vi "Triangle.vi"() -> ()   [LabVIEW 2017]
panel:
  out "Numeric":i32
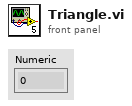
[diagram p1: front panel]
types:
  T1 = enum16{"Full", "Half", "Quarter", "Eighth", "Sixteenth"}
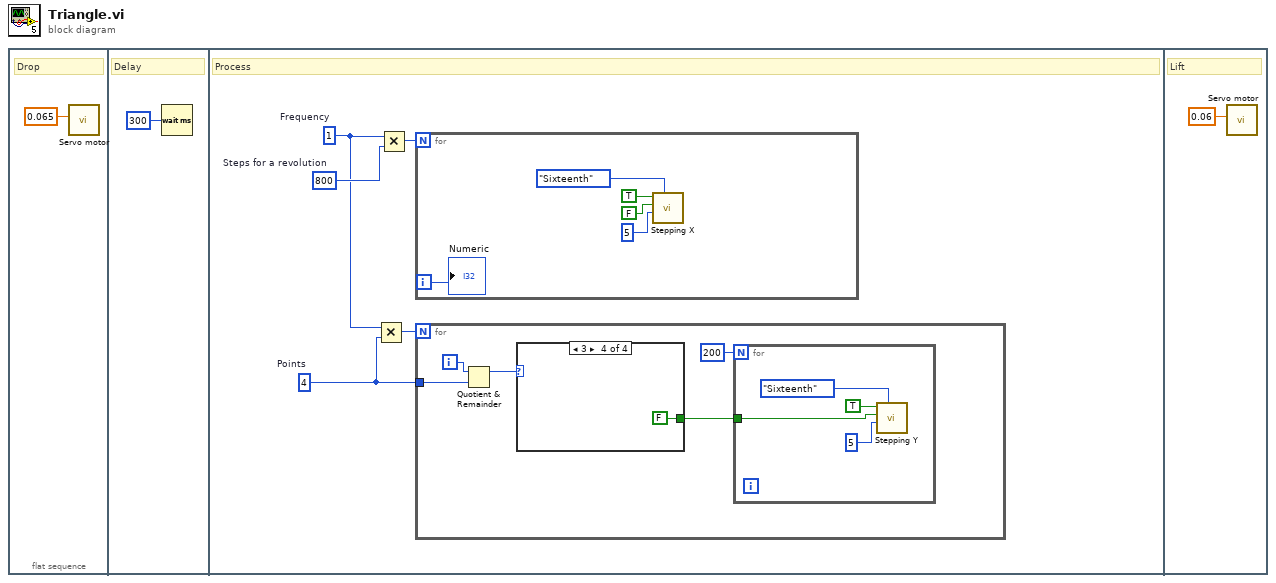
[diagram p0: block diagram]
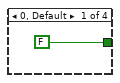
[diagram p2: hidden frame]
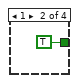
[diagram p3: hidden frame]
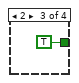
[diagram p4: hidden frame]
diagram:
  n1 = flat-sequence {
    frame #0 {
      # "Drop"
      n2 = call "Servo motor.vi"("Duty Cycle"=0.065) -> ()  [unwired: 9 in, 2 out]
    }
    frame #1 {
      # "Delay"
      n3 = Wait (ms)(milliseconds to wait=u32 300) -> ()  [unwired: 1 out]
    }
    frame #2 {
      w3 = 4  # Points
      w4 = 1  # Frequency
      w5 = 800  # Steps for a revolution
      # "Process"
      n4 = Multiply(x=w4, y=w3) -> (x*y=w7:i32)
      n5 = Multiply(x=w4, y=w5) -> (x*y=w6:i32)
      n6 = for {
        N: w6 -> [_]
        i -> [w25]
        n7 = call "Stepping X.vi"("Microstep size"=T1."Sixteenth", "Speed"=u32 5, "Direction"=FALSE, "Enable"=TRUE) -> ()  [unwired: 7 in, 1 out]
        "Numeric" <- w25
      }
      n8 = for {
        N: w7 -> [_]
        tunnel: w3 -> [w11]
        i -> [w12]
        n9 = Quotient & Remainder(x=w12, y=w11) -> (x-y*floor(x/y)=w10:i32)  [unwired: 1 out]
        n10 = case shown="3" w10 {
          tunnel: [FALSE ("Direction") TRUE ("Direction") TRUE ("Direction") FALSE ("Direction")] -> w9
          frame 0, Default {
          }
          frame 1 {
          }
          frame 2 {
          }
          frame 3 {
          }
        }
        n11 = for {
          N: 200 -> [_]
          tunnel: w9 -> [w13]
          n12 = call "Stepping Y.vi"("Microstep size"=T1."Sixteenth", "Speed"=u32 5, "Direction"=w13, "Enable"=TRUE) -> ()  [unwired: 7 in, 1 out]
        }
      }
    }
    frame #3 {
      # "Lift"
      n13 = call "Servo motor.vi"("Duty Cycle"=0.06) -> ()  [unwired: 9 in, 2 out]
    }
  }
